vi "cDAQ Digitizing Process.vi"(8 "error in":errorcluster, 11 "cdaq session":variant) -> (0 "error out":errorcluster)   [LabVIEW 2020]
uses:
  cDAQ Session.ctl
  low_level_old/cdaq_anal_adc_command.ctl
  low_level_old/cdaq_anal_adc_data.ctl
  cDAQ Virtual Channel.ctl
  cDAQ Master Clock Mode.ctl
  <vilib>/DAQmx/read.llb/DAQmx Read (Analog 2D DBL NChan NSamp).vi
  <vilib>/DAQmx/miscellaneous.llb/DAQmx Fill In Error Info.vi
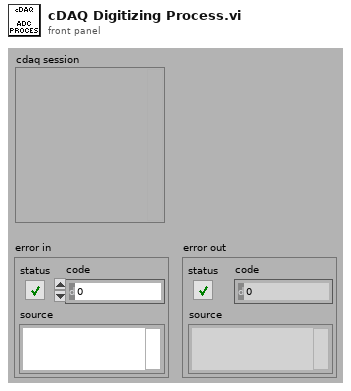
[diagram p1: front panel]
types:
  T1 = typedef "cDAQ Session.ctl" = cluster{"mclk [Hz]":dbl, "ADC task":refnum<k21>, "mclk reference":string, "fs [Hz]":dbl, "queue adc cmd":refnum<queue>, "queue adc data":refnum<queue>, "adc proc ref":refnum<vi>, "channels":T2[], "last channels":T2[], "timeout":timestamp, "N":i32, "mclk mode":T3, "ext mclk source":tag}
  T2 = typedef "cDAQ Virtual Channel.ctl" = cluster{"Device":tag, "Channel id":i32, "btn clr":bool, "btn up":bool, "btn down":bool}
  T3 = typedef "cDAQ Master Clock Mode.ctl" = enum16{"Free running", "Export master clock", "Import master clock"}
  T4 = typedef "cdaq_anal_adc_data.ctl" = cluster{"wave":dbl[][], "timestamp [s]":dbl, "abs timestamp":timestamp, "Aborted":bool}
  T5 = typedef "cdaq_anal_adc_command.ctl" = cluster{"sample to get":i32, "stop":bool, "abort":bool}
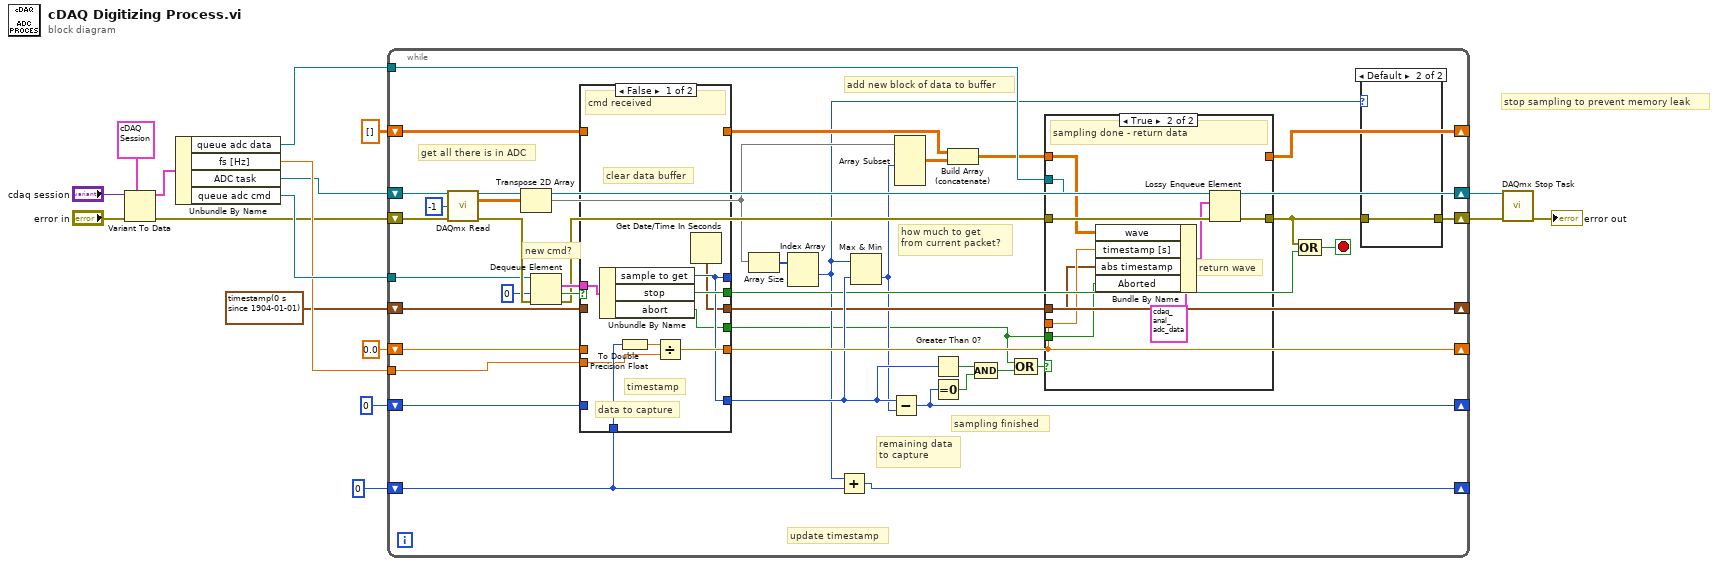
[diagram p0: block diagram]
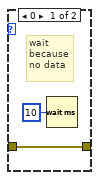
[diagram p2: hidden frame]
diagram:
  # "stop sampling to prevent memory leak"
  n1 = Variant To Data(error in="error in", type=T1 {"mclk [Hz]"=0.0, "ADC task"="", "mclk reference"="", "fs [Hz]"=50000.0, "queue adc cmd"=refnum, "queue adc data"=refnum, "adc proc ref"=refnum, "channels"=[], "last channels"=[], "timeout"=timestamp(0 s since 1904-01-01), "N"=0, "mclk mode"=enum."Free running", "ext mclk source"=""} ("cdaq session"), Variant="cdaq session") -> (data=w14:T1, error out=w3:errorcluster)
  n2 = Unbundle By Name(w14) -> ("queue adc data"=w8:refnum<queue>, "fs [Hz]"=w9:dbl, "ADC task"=w2:refnum<k21>, "queue adc cmd"=w13:refnum<queue>)
  n3 = while {
    shift-right: [w29] -> w6
    shift-left: w3 -> [w57]
    shift-right: [w39] -> w4
    shift-left: w2 -> [w56]
    shift-right: [w45] -> _
    shift-left: i64 0 -> [w47]
    tunnel: w13 -> [w53]
    shift-right: [w42] -> _
    shift-left: 0 -> [w34]
    shift-right: [w32] -> _
    shift-left: dbl[][] [] -> [w44]
    shift-right: [w36] -> _
    shift-left: 0.0 -> [w26]
    tunnel: w9 -> [w46]
    tunnel: w8 -> [w37]
    shift-right: [w25] -> _
    shift-left: timestamp(0 s since 1904-01-01) ("seconds since 1Jan1904") -> [w24]
    stop <- w30 stop-if-true
    # "new cmd?"
    # "get all there is in ADC"
    # "sampling finished"
    # "update timestamp"
    # "add new block of data to buffer"
    # "remaining data\nto capture"
    # "how much to get\nfrom current packet?"
    n4 = call-poly <vilib>:"DAQmx Read.vi"("task/channels in"=w56, "number of samples per channel"=-1, "error in"=w57) -> ("task out"=w39:refnum<k21>, "data"=w49:dbl[][], "error out"=w54:errorcluster)  [unwired: 10 in]
    n5 = Transpose 2D Array(2D array=w49) -> (transposed array=w23:dbl[][])
    n6 = Dequeue Element(queue=w53, timeout in ms (-1)=0, error in (no error)=w54) -> (element=w51:T5, timed out?=w50:bool, error out=w38:errorcluster)  [unwired: 1 out]
    n7 = case shown="False" w50 {
      tunnel: w51 -> [w80 _]
      tunnel: [w79 _] -> w31
      tunnel: [w74 _] -> _
      tunnel: w47 -> [w78 _]
      tunnel: w46 -> [w76 _]
      tunnel: [w75 w82] -> w36
      tunnel: [_ w84] -> w43
      tunnel: w44 -> [_ w84]
      tunnel: [w74 w83] -> w33
      tunnel: w34 -> [_ w83]
      tunnel: w26 -> [_ w82]
      tunnel: [w73 w81] -> w25
      tunnel: w24 -> [_ w81]
      tunnel: [w72 _] -> w18
      frame False {
        # "data to capture"
        # "clear data buffer"
        # "timestamp"
        # "cmd received"
        n8 = Unbundle By Name(w80) -> ("sample to get"=w74:i32, "stop"=w79:bool, "abort"=w72:bool)
        n9 = To Double Precision Float(number=w78) -> (double precision float=w77:dbl)
        n10 = Divide(x=w77, y=w76) -> (x/y=w75:dbl)
        n11 = Get Date/Time In Seconds() -> (seconds since 1Jan1904=w73:timestamp)
      }
      frame True {
        # "timeout"
      }
    }
    n12 = Array Size(array=w23) -> (size(s)=w27:i32[])
    n13 = Index Array(array=w27) -> (element #1=w21:i32)  [unwired: 2 in, 1 out]
    n14 = Add(x=w21, y=w47) -> (x+y=w45:i64)
    n15 = Max & Min(x=w21, y=w33) -> (min(x,y)=w22:i32)  [unwired: 1 out]
    n16 = Subtract(x=w33, y=w22) -> (x-y=w42:i32)
    n17 = Array Subset(array=w23, length (row)=w22) -> (w48:dbl[][])  [unwired: 3 in]
    n18 = Greater Than 0?(x=w33) -> (x > 0?=w41:bool)
    n19 = Equal To 0?(x=w42) -> (x = 0?=w40:bool)
    n20 = Build Array (concatenate)(w43, w48) -> (w35:dbl[][])
    n21 = Compound Arithmetic op=AND(w41, w40) -> (w20:bool)
    n22 = Compound Arithmetic op=OR(w18, w20) -> (w19:bool)
    n23 = case shown="True" w19 {
      tunnel: w38 -> [w61 w71]
      tunnel: w37 -> [_ w70]
      tunnel: w36 -> [_ w68]
      tunnel: w35 -> [w62 w66]
      tunnel: [w62 _] -> w32
      tunnel: [w61 w65] -> w28
      tunnel: w25 -> [_ w64]
      tunnel: w18 -> [_ w63]
      frame False {
      }
      frame True {
        # "return wave"
        # "sampling done - return data"
        n24 = Bundle By Name(cluster=T4 {"wave"=[], "timestamp [s]"=0.0, "abs timestamp"=timestamp(0 s since 1904-01-01), "Aborted"=FALSE} ("adc data"), "wave"=w66, "timestamp [s]"=w68, "abs timestamp"=w64, "Aborted"=w63) -> (w67:T4)
        n25 = Lossy Enqueue Element(queue=w70, element=w67, error in (no error)=w71) -> (error out=w65:errorcluster)  [unwired: 3 out]
      }
    }
    n26 = Compound Arithmetic op=OR(w28, w31) -> (w30:bool)
    n27 = case shown="Default" w21 {
      tunnel: [w59 w60] -> w29
      tunnel: w28 -> [w59 w60]
      frame 0 {
        # "wait\nbecause\nno data"
        n28 = Wait (ms)(milliseconds to wait=u32 10) -> ()  [unwired: 1 out]
      }
      frame Default {
      }
    }
  }
  n29 = call <vilib>:"DAQmx Stop Task.vi"("task/channels in"=w4, "error in"=w6) -> ("error out"=→"error out":errorcluster)  [unwired: 12 in, 1 out]
